vi "XML Read Value.vi"(6 "Default Attribute Values":variant[](array[variant]), 7 "Attribute Names":string[](array[string]), 8 "error in (no error)":errorcluster, 9 "Default Element Value":variant, 10 "Element Name":string, 11 "XML Reader In":T1) -> (0 "error out":errorcluster, 1 "Element Value":variant, 2 "Found?":bool, 3 "XML Reader Out":T1, 4 "Attribute Values":variant[](array[variant]))   [LabVIEW 2016, in "Pathloss XML Reader.lvlib"]
uses:
  Pathloss XML Reader.lvlib
  Controls/XML Reader Data Ref.ctl
  Controls/XML Reader Data.ctl
  <vilib>/Utility/VariantDataType/VariantType.lvlib
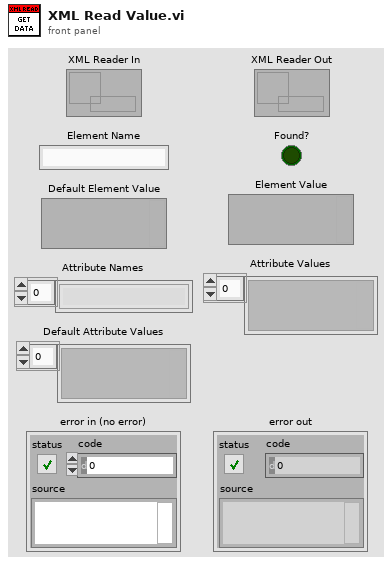
[diagram p1: front panel]
types:
  T1 = typedef "Pathloss XML Reader.lvlib/XML Reader Data Ref.ctl" = refnum<data-value>
  T2 = typedef "Pathloss XML Reader.lvlib/XML Reader Data.ctl" = cluster{"Remaining XML":string, "Section Name Stack":string[], "Section Stack":string[]}
  T3 = typedef "VariantType.lvlib/Type.ctl" = enum8{"Invalid Type", "Void", "I8", "I16", "I32", "I64", "U8", "U16", "U32", "U64", "Single Float", "Double Float", "Extended Float", "Single Complex", "Double Complex", "Extended Complex", "Enum U8", "Enum U16", "Enum U32", "Enum U64", "Single Float With Unit", "Double Float With Unit", "Extended Float With Unit", "Single Complex with Unit", "Double Complex with Unit", "Extended Complex with Unit", "Boolean", "String", "Path", "Picture", "Tag", "Array", "Cluster", "Variant", "LV Variant", "Waveform", "Timestamp", "Digital Waveform", "Digital Data", "ExpressData", "Refnum", "External Data", "VI", "Poly VI", "LabVIEW Class Instance", "Fixed Point"}
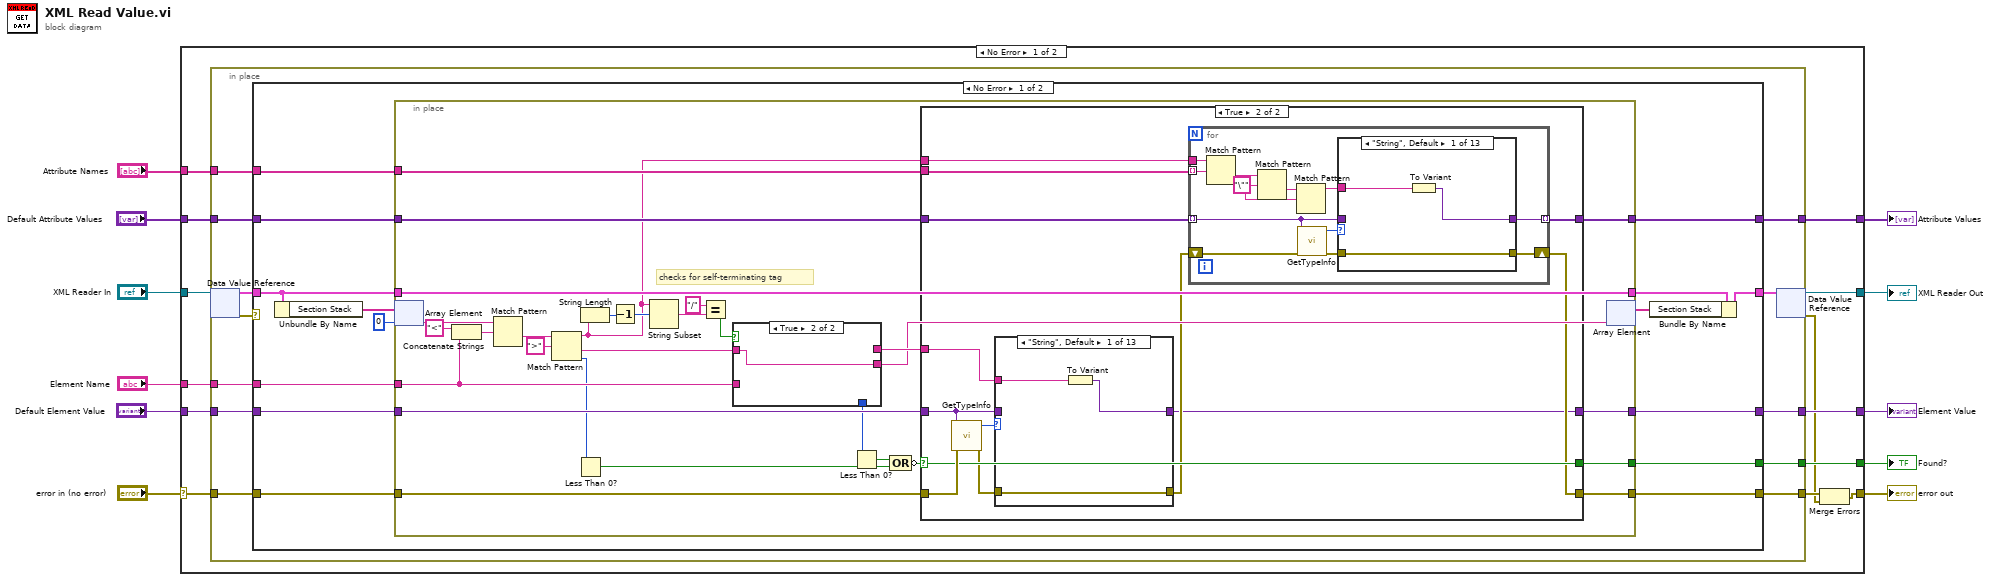
[diagram p0: block diagram]
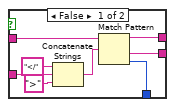
[diagram p2: hidden frame]
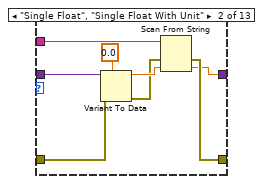
[diagram p4: hidden frame]
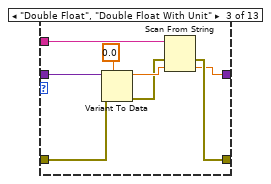
[diagram p5: hidden frame]
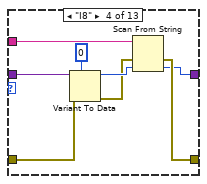
[diagram p6: hidden frame]
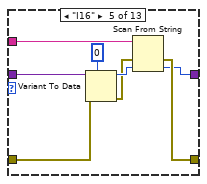
[diagram p7: hidden frame]
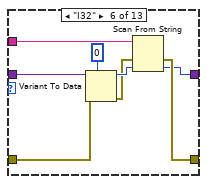
[diagram p8: hidden frame]
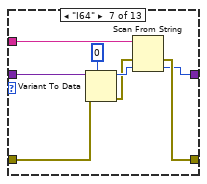
[diagram p9: hidden frame]
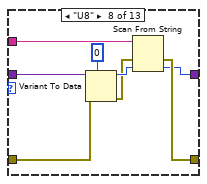
[diagram p10: hidden frame]
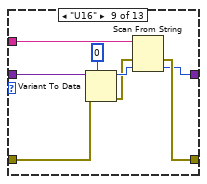
[diagram p11: hidden frame]
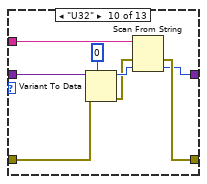
[diagram p12: hidden frame]
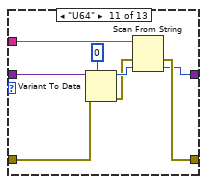
[diagram p13: hidden frame]
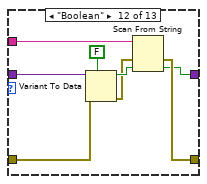
[diagram p14: hidden frame]
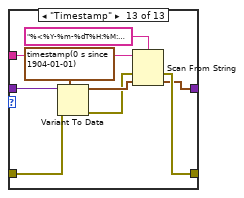
[diagram p15: hidden frame]
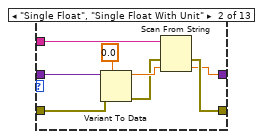
[diagram p16: hidden frame]
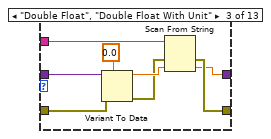
[diagram p17: hidden frame]
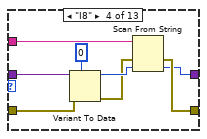
[diagram p18: hidden frame]
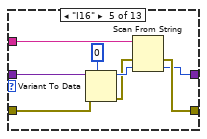
[diagram p19: hidden frame]
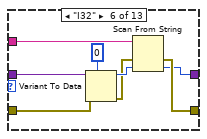
[diagram p20: hidden frame]
diagram:
  n1 = case shown="No Error" "error in (no error)" {
    selector: "error in (no error)" -> [w22 w325]
    tunnel: [w13 w325] -> w10
    tunnel: [w23 w326] -> w9
    tunnel: "XML Reader In" -> [w24 w326]
    tunnel: "Element Name" -> [w20 _]
    tunnel: "Attribute Names" -> [w19 _]
    tunnel: "Default Attribute Values" -> [w18 w324]
    tunnel: "Default Element Value" -> [w17 w323]
    tunnel: [w16 _] -> w1
    tunnel: [w15 w324] -> w4
    tunnel: [w14 w323] -> w2
    frame No Error {
      n2 = in-place {
        in-place-border: w22 -> [w33]
        in-place-border: [w32] -> w21
        in-place-border: w20 -> [w31]
        in-place-border: w19 -> [w30]
        in-place-border: w18 -> [w29]
        in-place-border: w17 -> [w28]
        in-place-border: [w27] -> w16
        in-place-border: [w26] -> w15
        in-place-border: [w25] -> w14
        n3 = in-place-dvr #1(w24) -> (w35:T2, w36:errorcluster)
        n4 = case shown="No Error" w36 {
          selector: w36 -> [_ w321]
          tunnel: w35 -> [w39 w322]
          tunnel: [w38 w322] -> w34
          tunnel: w33 -> [w51 _]
          tunnel: [w50 w321] -> w32
          tunnel: w31 -> [w48 _]
          tunnel: w30 -> [w44 _]
          tunnel: w29 -> [w45 w320]
          tunnel: w28 -> [w47 w319]
          tunnel: [w46 _] -> w27
          tunnel: [w43 w320] -> w26
          tunnel: [w42 w319] -> w25
          frame No Error {
            n5 = Unbundle By Name(w39) -> ("Section Stack"=w41:string[])
            n6 = in-place {
              in-place-border: w51 -> [w74]
              in-place-border: [w73] -> w50
              in-place-border: [w58] -> w49
              in-place-border: w48 -> [w70]
              in-place-border: w47 -> [w69]
              in-place-border: [w66] -> w46
              in-place-border: w45 -> [w65]
              in-place-border: w44 -> [w64]
              in-place-border: [w63] -> w43
              in-place-border: [w62] -> w42
              in-place-border: w39 -> [w58]
              # "checks for self-terminating tag"
              n7 = in-place-array #2(w41, 0) -> (w60:string)
              n8 = Concatenate Strings("<" ("string"), w70) -> (w79:string)
              n9 = Match Pattern(string=w60, regular expression=w79) -> (after substring=w78:string)  [unwired: 1 in, 3 out]
              n10 = Match Pattern(string=w78, regular expression=">") -> (before substring=w55:string, after substring=w72:string, offset past match=w67:i32)  [unwired: 1 in, 1 out]
              n11 = Less Than 0?(x=w67) -> (x < 0?=w76:bool)
              n12 = String Length(string=w55) -> (length=w57:i32)
              n13 = Decrement(x=w57) -> (x-1=w56:i32)
              n14 = String Subset(string=w55, offset (0)=w56) -> (substring=w54:string)  [unwired: 1 in]
              n15 = Equal?(x="/", y=w54) -> (x = y?=w52:bool)
              n16 = case shown="True" w52 {
                tunnel: w72 -> [w88 w89]
                tunnel: w70 -> [w85 _]
                tunnel: [w83 _] -> w68
                tunnel: [w82 _] -> w61
                tunnel: [w81 w89] -> w59
                frame False {
                  n17 = Concatenate Strings("</" ("string"), w85, ">" ("string")) -> (w84:string)
                  n18 = Match Pattern(string=w88, regular expression=w84) -> (before substring=w82:string, after substring=w81:string, offset past match=w83:i32)  [unwired: 1 in, 1 out]
                }
                frame True {
                }
              }
              n19 = Less Than 0?(x=w68) -> (x < 0?=w71:bool)
              n20 = Compound Arithmetic op=OR(w71, w76) -> (invert w75:bool)
              n21 = case shown="True" w75 {
                selector: w75 -> [w92 w105]
                tunnel: w74 -> [w93 w106]
                tunnel: [w93 w101] -> w73
                tunnel: w69 -> [w90 w95]
                tunnel: w55 -> [_ w103]
                tunnel: w61 -> [_ w99]
                tunnel: [w92 w105] -> w66
                tunnel: w65 -> [w91 w102]
                tunnel: w64 -> [_ w104]
                tunnel: [w91 w100] -> w63
                tunnel: [w90 w94] -> w62
                frame False {
                }
                frame True {
                  n22 = call <vilib>:"GetTypeInfo.vi"("error in (no error)"=w106, "Variant"=w95) -> ("error out"=w97:errorcluster, "Type Enum"=w98:T3)  [unwired: 5 in, 3 out]
                  n23 = case shown="\"String\", Default" w98 {
                    tunnel: w99 -> [w108 w117 w125 w133 w141 w149 w157 w165 w173 w181 w189 w197 w206]
                    tunnel: w95 -> [_ w116 w124 w132 w140 w148 w156 w164 w172 w180 w188 w196 w205]
                    tunnel: w97 -> [w109 w115 w123 w131 w139 w147 w155 w163 w171 w179 w187 w195 w204]
                    tunnel: [w109 w112 w120 w128 w136 w144 w152 w160 w168 w176 w184 w192 w201] -> w96
                    tunnel: [w107 w110 w118 w126 w134 w142 w150 w158 w166 w174 w182 w190 w199] -> w94
                    frame "String", Default {
                      n24 = To Variant(anything=w108) -> (Variant=w107:variant)
                    }
                    frame "Single Float", "Single Float With Unit" {
                      n25 = Variant To Data(error in=w115, type=sgl 0.0, Variant=w116) -> (data=w114:sgl, error out=w113:errorcluster)
                      n26 = Scan From String(input string=w117, error in=w113, default 1=w114) -> (error out=w112:errorcluster, output 1=w110:sgl)  [unwired: 2 in, 2 out]
                    }
                    frame "Double Float", "Double Float With Unit" {
                      n27 = Variant To Data(error in=w123, type=0.0, Variant=w124) -> (data=w122:dbl, error out=w121:errorcluster)
                      n28 = Scan From String(input string=w125, error in=w121, default 1=w122) -> (error out=w120:errorcluster, output 1=w118:dbl)  [unwired: 2 in, 2 out]
                    }
                    frame "I8" {
                      n29 = Variant To Data(error in=w131, type=i8 0, Variant=w132) -> (data=w130:i8, error out=w129:errorcluster)
                      n30 = Scan From String(input string=w133, error in=w129, default 1=w130) -> (error out=w128:errorcluster, output 1=w126:i8)  [unwired: 2 in, 2 out]
                    }
                    frame "I16" {
                      n31 = Variant To Data(error in=w139, type=i16 0, Variant=w140) -> (data=w138:i16, error out=w137:errorcluster)
                      n32 = Scan From String(input string=w141, error in=w137, default 1=w138) -> (error out=w136:errorcluster, output 1=w134:i16)  [unwired: 2 in, 2 out]
                    }
                    frame "I32" {
                      n33 = Variant To Data(error in=w147, type=0, Variant=w148) -> (data=w146:i32, error out=w145:errorcluster)
                      n34 = Scan From String(input string=w149, error in=w145, default 1=w146) -> (error out=w144:errorcluster, output 1=w142:i32)  [unwired: 2 in, 2 out]
                    }
                    frame "I64" {
                      n35 = Variant To Data(error in=w155, type=i64 0, Variant=w156) -> (data=w154:i64, error out=w153:errorcluster)
                      n36 = Scan From String(input string=w157, error in=w153, default 1=w154) -> (error out=w152:errorcluster, output 1=w150:i64)  [unwired: 2 in, 2 out]
                    }
                    frame "U8" {
                      n37 = Variant To Data(error in=w163, type=u8 0, Variant=w164) -> (data=w162:u8, error out=w161:errorcluster)
                      n38 = Scan From String(input string=w165, error in=w161, default 1=w162) -> (error out=w160:errorcluster, output 1=w158:u8)  [unwired: 2 in, 2 out]
                    }
                    frame "U16" {
                      n39 = Variant To Data(error in=w171, type=u16 0, Variant=w172) -> (data=w170:u16, error out=w169:errorcluster)
                      n40 = Scan From String(input string=w173, error in=w169, default 1=w170) -> (error out=w168:errorcluster, output 1=w166:u16)  [unwired: 2 in, 2 out]
                    }
                    frame "U32" {
                      n41 = Variant To Data(error in=w179, type=u32 0, Variant=w180) -> (data=w178:u32, error out=w177:errorcluster)
                      n42 = Scan From String(input string=w181, error in=w177, default 1=w178) -> (error out=w176:errorcluster, output 1=w174:u32)  [unwired: 2 in, 2 out]
                    }
                    frame "U64" {
                      n43 = Variant To Data(error in=w187, type=u64 0, Variant=w188) -> (data=w186:u64, error out=w185:errorcluster)
                      n44 = Scan From String(input string=w189, error in=w185, default 1=w186) -> (error out=w184:errorcluster, output 1=w182:u64)  [unwired: 2 in, 2 out]
                    }
                    frame "Boolean" {
                      n45 = Variant To Data(error in=w195, type=FALSE, Variant=w196) -> (data=w194:bool, error out=w193:errorcluster)
                      n46 = Scan From String(input string=w197, error in=w193, default 1=w194) -> (error out=w192:errorcluster, output 1=w190:bool)  [unwired: 2 in, 2 out]
                    }
                    frame "Timestamp" {
                      n47 = Variant To Data(error in=w204, type=timestamp(0 s since 1904-01-01), Variant=w205) -> (data=w203:timestamp, error out=w202:errorcluster)
                      n48 = Scan From String(format string="%<%Y-%m-%dT%H:%M:%S%7u%z>T" ("regular expression"), input string=w206, error in=w202, default 1=w203) -> (error out=w201:errorcluster, output 1=w199:timestamp)  [unwired: 1 in, 2 out]
                    }
                  }
                  n49 = for {
                    tunnel: w103 -> [w218]
                    tunnel: w104 -> [w217] mode=indexing
                    tunnel: w102 -> [w210] mode=indexing
                    shift-right: [w208] -> w101
                    shift-left: w96 -> [w213]
                    tunnel: [w207] -> w100 mode=indexing
                    w214 = "\"" ("regular expression")
                    n50 = Match Pattern(string=w218, regular expression=w217) -> (after substring=w216:string)  [unwired: 1 in, 3 out]
                    n51 = Match Pattern(string=w216, regular expression=w214) -> (after substring=w215:string)  [unwired: 1 in, 3 out]
                    n52 = Match Pattern(string=w215, regular expression=w214) -> (before substring=w211:string)  [unwired: 1 in, 3 out]
                    n53 = call <vilib>:"GetTypeInfo.vi"("error in (no error)"=w213, "Variant"=w210) -> ("error out"=w209:errorcluster, "Type Enum"=w212:T3)  [unwired: 5 in, 3 out]
                    n54 = case shown="\"String\", Default" w212 {
                      tunnel: w211 -> [w220 w229 w237 w245 w253 w261 w269 w277 w285 w293 w301 w309 w318]
                      tunnel: w210 -> [_ w228 w236 w244 w252 w260 w268 w276 w284 w292 w300 w308 w317]
                      tunnel: w209 -> [w221 w227 w235 w243 w251 w259 w267 w275 w283 w291 w299 w307 w316]
                      tunnel: [w221 w224 w232 w240 w248 w256 w264 w272 w280 w288 w296 w304 w313] -> w208
                      tunnel: [w219 w222 w230 w238 w246 w254 w262 w270 w278 w286 w294 w302 w311] -> w207
                      frame "String", Default {
                        n55 = To Variant(anything=w220) -> (Variant=w219:variant)
                      }
                      frame "Single Float", "Single Float With Unit" {
                        n56 = Variant To Data(error in=w227, type=sgl 0.0, Variant=w228) -> (data=w226:sgl, error out=w225:errorcluster)
                        n57 = Scan From String(input string=w229, error in=w225, default 1=w226) -> (error out=w224:errorcluster, output 1=w222:sgl)  [unwired: 2 in, 2 out]
                      }
                      frame "Double Float", "Double Float With Unit" {
                        n58 = Variant To Data(error in=w235, type=0.0, Variant=w236) -> (data=w234:dbl, error out=w233:errorcluster)
                        n59 = Scan From String(input string=w237, error in=w233, default 1=w234) -> (error out=w232:errorcluster, output 1=w230:dbl)  [unwired: 2 in, 2 out]
                      }
                      frame "I8" {
                        n60 = Variant To Data(error in=w243, type=i8 0, Variant=w244) -> (data=w242:i8, error out=w241:errorcluster)
                        n61 = Scan From String(input string=w245, error in=w241, default 1=w242) -> (error out=w240:errorcluster, output 1=w238:i8)  [unwired: 2 in, 2 out]
                      }
                      frame "I16" {
                        n62 = Variant To Data(error in=w251, type=i16 0, Variant=w252) -> (data=w250:i16, error out=w249:errorcluster)
                        n63 = Scan From String(input string=w253, error in=w249, default 1=w250) -> (error out=w248:errorcluster, output 1=w246:i16)  [unwired: 2 in, 2 out]
                      }
                      frame "I32" {
                        n64 = Variant To Data(error in=w259, type=0, Variant=w260) -> (data=w258:i32, error out=w257:errorcluster)
                        n65 = Scan From String(input string=w261, error in=w257, default 1=w258) -> (error out=w256:errorcluster, output 1=w254:i32)  [unwired: 2 in, 2 out]
                      }
                      frame "I64" {
                        n66 = Variant To Data(error in=w267, type=i64 0, Variant=w268) -> (data=w266:i64, error out=w265:errorcluster)
                        n67 = Scan From String(input string=w269, error in=w265, default 1=w266) -> (error out=w264:errorcluster, output 1=w262:i64)  [unwired: 2 in, 2 out]
                      }
                      frame "U8" {
                        n68 = Variant To Data(error in=w275, type=u8 0, Variant=w276) -> (data=w274:u8, error out=w273:errorcluster)
                        n69 = Scan From String(input string=w277, error in=w273, default 1=w274) -> (error out=w272:errorcluster, output 1=w270:u8)  [unwired: 2 in, 2 out]
                      }
                      frame "U16" {
                        n70 = Variant To Data(error in=w283, type=u16 0, Variant=w284) -> (data=w282:u16, error out=w281:errorcluster)
                        n71 = Scan From String(input string=w285, error in=w281, default 1=w282) -> (error out=w280:errorcluster, output 1=w278:u16)  [unwired: 2 in, 2 out]
                      }
                      frame "U32" {
                        n72 = Variant To Data(error in=w291, type=u32 0, Variant=w292) -> (data=w290:u32, error out=w289:errorcluster)
                        n73 = Scan From String(input string=w293, error in=w289, default 1=w290) -> (error out=w288:errorcluster, output 1=w286:u32)  [unwired: 2 in, 2 out]
                      }
                      frame "U64" {
                        n74 = Variant To Data(error in=w299, type=u64 0, Variant=w300) -> (data=w298:u64, error out=w297:errorcluster)
                        n75 = Scan From String(input string=w301, error in=w297, default 1=w298) -> (error out=w296:errorcluster, output 1=w294:u64)  [unwired: 2 in, 2 out]
                      }
                      frame "Boolean" {
                        n76 = Variant To Data(error in=w307, type=FALSE, Variant=w308) -> (data=w306:bool, error out=w305:errorcluster)
                        n77 = Scan From String(input string=w309, error in=w305, default 1=w306) -> (error out=w304:errorcluster, output 1=w302:bool)  [unwired: 2 in, 2 out]
                      }
                      frame "Timestamp" {
                        n78 = Variant To Data(error in=w316, type=timestamp(0 s since 1904-01-01), Variant=w317) -> (data=w315:timestamp, error out=w314:errorcluster)
                        n79 = Scan From String(format string="%<%Y-%m-%dT%H:%M:%S%7u%z>T" ("regular expression"), input string=w318, error in=w314, default 1=w315) -> (error out=w313:errorcluster, output 1=w311:timestamp)  [unwired: 1 in, 2 out]
                      }
                    }
                  }
                }
              }
              n80 = in-place-array #2(w59) -> (w37:string[])  [unwired: 1 out]
            }
            n81 = Bundle By Name(cluster=w49, "Section Stack"=w37) -> (w38:T2)
          }
          frame Error {
          }
        }
        n82 = in-place-dvr #1(w34) -> (w23:T1, w12:errorcluster)
      }
      n83 = Merge Errors(w21, w12) -> (w13:errorcluster)
    }
    frame Error {
    }
  }
  "error out" <- w10
  "XML Reader Out" <- w9
  "Element Value" <- w2
  "Attribute Values" <- w4
  "Found?" <- w1
